vi "Untitled 2.vi"(8 "error in (no error)":errorcluster, 11 "EditPanel API in":refnum<class "EditPanel API.lvclass">) -> (0 "error out":errorcluster, 3 "EditPanel API out":refnum<class "EditPanel API.lvclass">)   [LabVIEW 2015]
uses:
  EditPanel API.lvclass
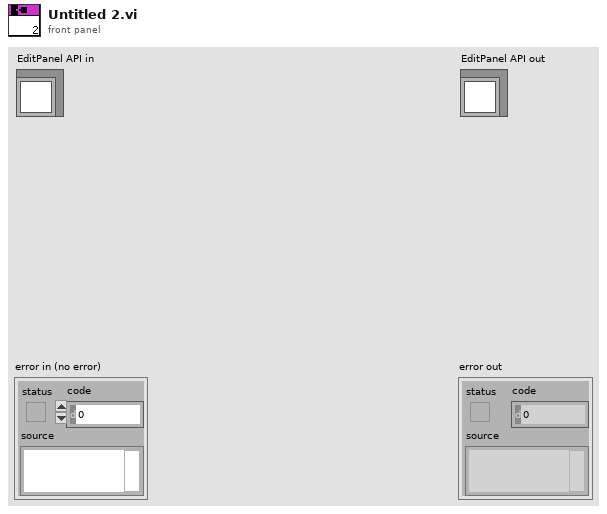
[diagram p1: front panel]
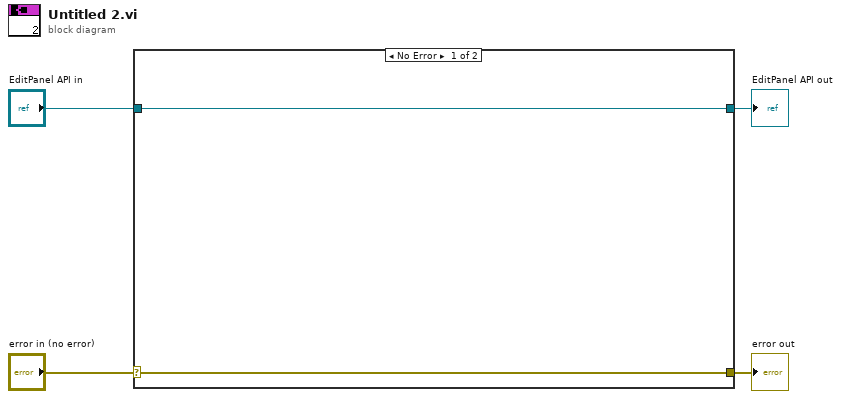
[diagram p0: block diagram]
diagram:
  n1 = case shown="No Error" "error in (no error)" {
    selector: "error in (no error)" -> [w5 w8]
    tunnel: [w5 w8] -> w3
    tunnel: [w6 w7] -> w1
    tunnel: "EditPanel API in" -> [w6 w7]
    frame No Error {
    }
    frame Error {
    }
  }
  "error out" <- w3
  "EditPanel API out" <- w1
